vi "Query Period.vi"(6 "channel":i32=1 min=1 max=4, 8 "error in (no error)":errorcluster, 11 "VISA resource name":refnum<visa-resource-name>) -> (0 "error Out (no error)":errorcluster, 2 "period (s)":i64, 3 "VISA resource name out":refnum<visa-resource-name>)   [LabVIEW 2019, in "Pulse Rider PG-1000.lvlib"]
doc: "Query the number of cycles (burst count) to be output in burst mode for the specified output channel.\n\ncycles number: the number of repetitions for each burst\nchannel: the output channel int from 1 to 4"
uses:
  <instrlib>/LV_PulseRiderPG1000/Pulse Rider PG-1000.lvlib
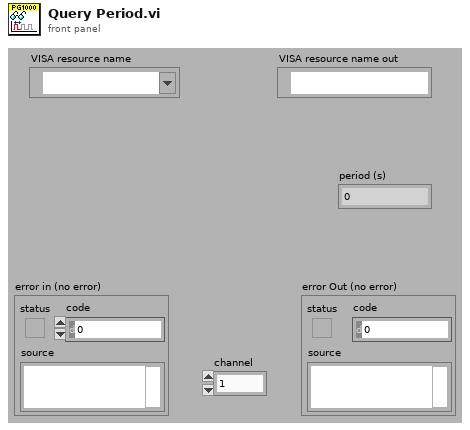
[diagram p1: front panel]
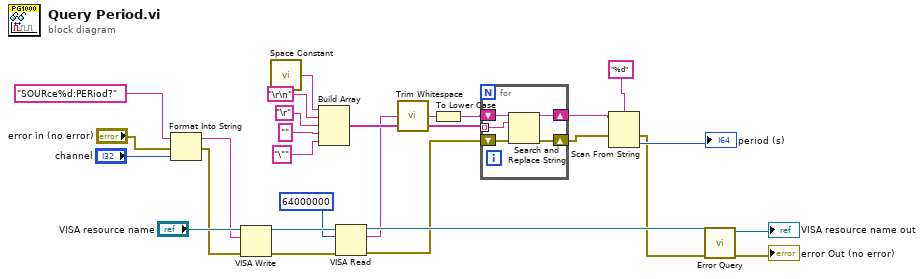
[diagram p0: block diagram]
diagram:
  n1 = Format Into String(format string="SOURce%d:PERiod?", error in="error in (no error)", "channel") -> (resulting string=w9:string, error out=w2:errorcluster)  [unwired: 1 in]
  n2 = VISA Write(VISA resource name="VISA resource name", write buffer=w9, error in (no error)=w2) -> (VISA resource name out=w24:refnum<visa-resource-name>, error out=w23:errorcluster)  [unwired: 1 out]
  n3 = call <vilib>:"Space Constant.vi"() -> ("String"=w20:string)
  n4 = Build Array(w20, "\r\n", "\r", "", "\"") -> (w15:string[])
  n5 = VISA Read(VISA resource name=w24, byte count=u32 64000000, error in (no error)=w23) -> (VISA resource name out=w21:refnum<visa-resource-name>, read buffer=w13:string, error out=w4:errorcluster)  [unwired: 1 out]
  n6 = call <vilib>:"Trim Whitespace.vi"("string"=w13) -> ("trimmed string"=w14:string)  [unwired: 1 in]
  n7 = To Lower Case(string=w14) -> (all lower case string=w12:string)
  n8 = for {
    tunnel: w15 -> [w30] mode=indexing
    shift-right: [w32] -> w8
    shift-left: w12 -> [w31]
    shift-right: [w28] -> w3
    shift-left: w4 -> [w29]
    n9 = Search and Replace String(input string=w31, search string=w30, error in=w29) -> (result string=w32:string, error out=w28:errorcluster)  [unwired: 5 in, 2 out]
  }
  n10 = Scan From String(format string="%d", input string=w8, error in=w3) -> (error out=w5:errorcluster, output 1=→"period (s)":i64)  [unwired: 2 in, 2 out]
  n11 = call <instrlib>:"Error Query.vi"("error in (no error)"=w5, "VISA resource name"=w21) -> ("error out"=→"error Out (no error)":errorcluster, "VISA resource name out"=→"VISA resource name out":refnum<visa-resource-name>)  [unwired: 6 in, 2 out]
